vi "IHM_cartoVisualization.vi"() -> ()   [LabVIEW 2009]
uses:
  <vilib>/Utility/miscctls.llb/LVRectTypeDef.ctl
panel:
  in  "Limites de la zone de tracé":T1
  in  "stop":bool
  in  "Nbr. Colonnes":i16
  in  "Nbr. Lignes":i16
  out "Carto signal":dbl[][](graph)
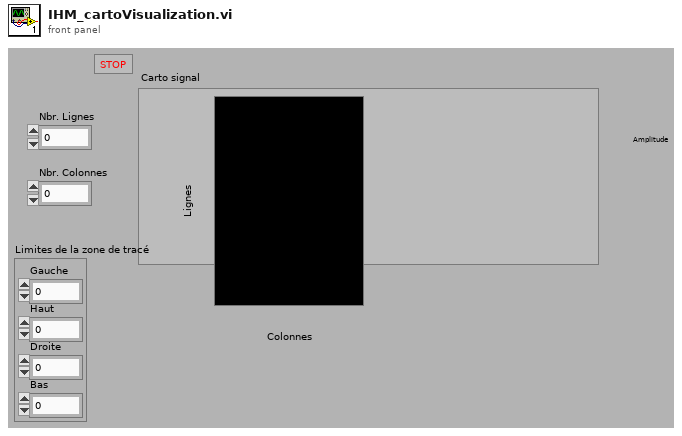
[diagram p1: front panel]
types:
  T1 = typedef "LVRectTypeDef.ctl" = cluster{"Left":i16, "Top":i16, "Right":i16, "Bottom":i16}
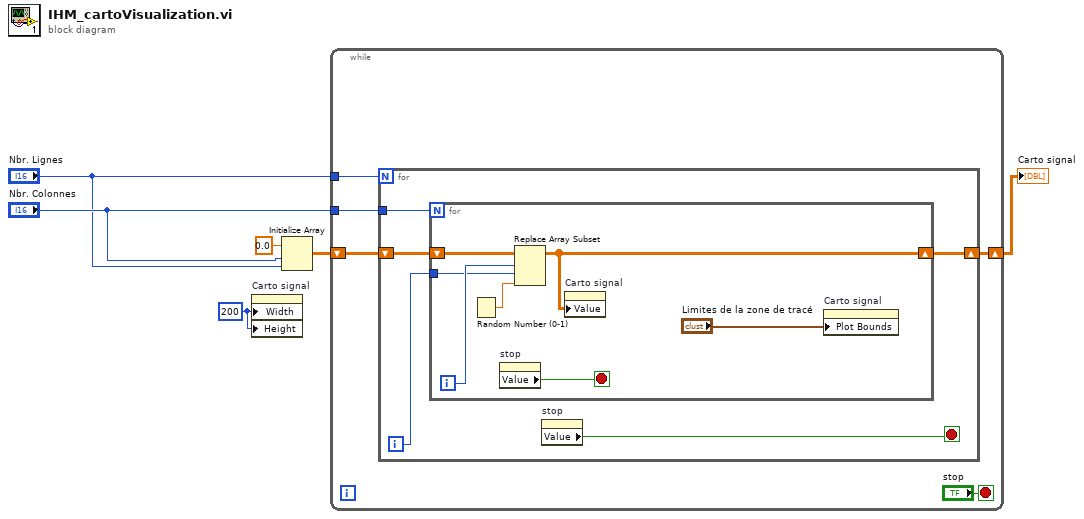
[diagram p0: block diagram]
diagram:
  w1 = u32 200 ("Zone de tracé : taille : largeur")
  n1 = property on="Carto signal" class="GraphInt (strict)"("Width"=w1, "Height"=w1) -> ()  [unwired: 2 in, 2 out]
  n2 = Initialize Array(0.0 ("élément"), "Nbr. Colonnes", "Nbr. Lignes") -> (w5:dbl[][])
  n3 = while {
    tunnel: "Nbr. Lignes" -> [w10]
    tunnel: "Nbr. Colonnes" -> [w9]
    shift-right: [w7] -> w4
    shift-left: w5 -> [w8]
    stop <- "stop" stop-if-true
    n4 = for {
      N: w10 -> [_]
      tunnel: w9 -> [w16]
      shift-right: [w12] -> w7
      shift-left: w8 -> [w14]
      i -> [w13]
      stop <- w15 stop-if-true
      n5 = for {
        N: w16 -> [_]
        tunnel: w13 -> [w18]
        shift-right: [w21] -> w12
        shift-left: w14 -> [w22]
        i -> [w19]
        stop <- w23 stop-if-true
        n6 = Random Number (0-1)() -> (number: 0 to 1=w20:dbl)
        n7 = property on="stop" class="Bool (strict)"() -> ("Value"=w23:bool)  [unwired: 2 in, 2 out]
        n8 = Replace Array Subset(array=w22, new element=w20, index (row)=w19, index (col)=w18) -> (w21:dbl[][])
        n9 = property on="Carto signal" class="GraphInt (strict)"("Value"=w21) -> ()  [unwired: 2 in, 2 out]
        n10 = property on="Carto signal" class="GraphInt (strict)"("Plot Bounds"="Limites de la zone de tracé") -> ()  [unwired: 2 in, 2 out]
      }
      n11 = property on="stop" class="Bool (strict)"() -> ("Value"=w15:bool)  [unwired: 2 in, 2 out]
    }
  }
  "Carto signal" <- w4
